vi "jettl Msg Last Ack Created Event.vi"(10 "Event":refnum<class "Event.lvclass">) -> (2 "Msg Strategy":refnum<class "Msg Strategy.lvclass">)   [LabVIEW 2021, in "jettl.lvlib" / "Last Ack Created Event Msg Strategy.lvlib"]
uses:
  Last Ack Created Event Msg Strategy.lvlib
  Event/Event.lvclass
  Msg Strategy/Msg Strategy.lvclass
  Last Ack Created Event Msg Strategy/Last Ack Created Event Msg Strategy.lvclass
  C:/git/jettl/jettl/jettl/Msg Strategy/Msg Strategy.lvclass
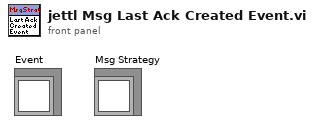
[diagram p1: front panel]
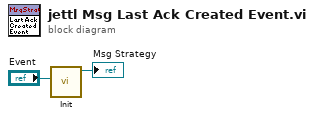
[diagram p0: block diagram]
diagram:
  n1 = call "Init.vi"("Event"="Event") -> ("Last Ack Created Event Msg Strategy out"=→"Msg Strategy":refnum<class "Last Ack Created Event Msg Strategy.lvclass">)  [unwired: 10 in]
